vi "Cleanup Session.vi"(8 "error in":errorcluster, 11 "Plugin in":refnum<class "Spectrogram.lvclass">) -> (0 "error out":errorcluster, 3 "Plugin out":refnum<class "Spectrogram.lvclass">)   [LabVIEW 2023, in "Spectrogram.lvlib" / "Spectrogram.lvclass"]
uses:
  Spectrogram.lvclass
  Spectrogram.lvclass/Spectrogram.ctl
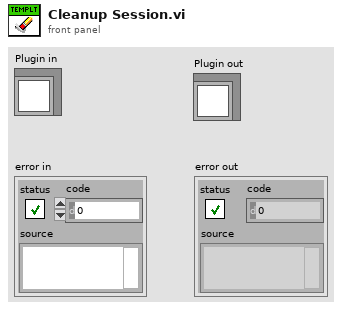
[diagram p1: front panel]
types:
  T1 = enum32{"Invalid", "Standard", "Closed", "Hidden", "Minimized", "Maximized"}
  T2 = typedef "Spectrogram.lvlib/Spectrogram.lvclass/Spectrogram Data.ctl" = cluster{"First Time":bool, "Show Spectrogram Window":bool, "Show Spectrogram Window Button Clicked":bool, "Extension":u16, "Time steps":i32, "Frequency bins":i32, "Type":i32, "Length":i32, "Color Table":u16, "Spectrogram VI Ref":refnum<vi>}
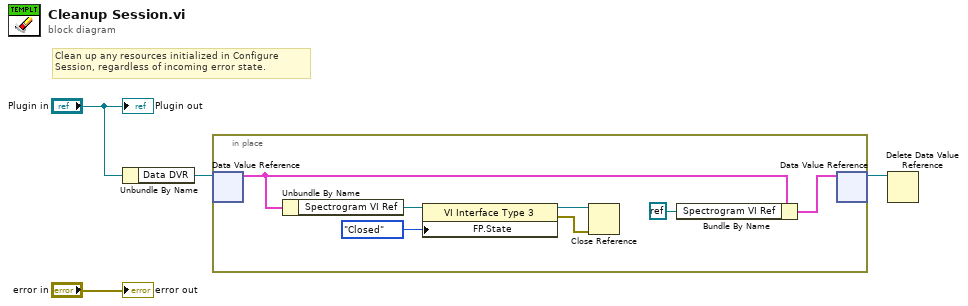
[diagram p0: block diagram]
diagram:
  # "Clean up any resources initialized in Configure Session, regardless of incoming error state."
  n1 = Unbundle By Name("Plugin in") -> ("Data DVR"=w3:refnum<data-value>)
  n2 = in-place {
    n3 = in-place-dvr #1(w3) -> (w11:T2)  [unwired: 1 out]
    n4 = Unbundle By Name(w11) -> ("Spectrogram VI Ref"=w8:refnum<vi>)
    n5 = property class="VI Interface Type 3"(reference=w8, "FP.State"=T1."Closed" ("Front Panel Window:State")) -> (reference out=w7:refnum<vi>, error out=w5:errorcluster)  [unwired: 1 in]
    n6 = Close Reference(reference=w7, error in (no error)=w5) -> ()  [unwired: 1 out]
    n7 = Bundle By Name(cluster=w11, "Spectrogram VI Ref"=refnum<k0> refnum) -> (w9:T2)
    n8 = in-place-dvr #1(w9) -> (w2:refnum<data-value>)  [unwired: 1 out]
  }
  n9 = Delete Data Value Reference(data value reference=w2) -> ()  [unwired: 1 in, 2 out]
  "error out" <- "error in"
  "Plugin out" <- "Plugin in"
